vi "LEDColorControlRob.vi"(8 "error in":errorcluster) -> ()   [LabVIEW 2014]
uses:
  <vilib>/Rock Robotics/WPI/DriverStation/WPI_DriverStationRobotMode2.ctl
  <vilib>/Rock Robotics/WPI/Joystick/WPI_JoystickGetSetRefNum.vi
  Gantry/GantryGlobals.vi
  Robot Global Data.vi
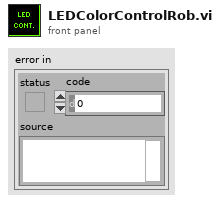
[diagram p1: front panel]
types:
  T1 = typedef "WPI_DriverStationRobotMode2.ctl" = enum16{"Autonomous Disabled", "Autonomous Enabled", "Teleop Disabled", "Teleop Enabled", "Disconnected", "Finish", "Test Disabled", "Test Enabled", "Emergency Stopped"}
  T2 = typedef "WPI_SPIDevRef.ctl" = cluster{"DevStatus":errorcluster, "Handle":i32, "Controller":T3, "SPI Bus":T4}
  T3 = typedef "FPGA_TypedefDigitalModule.ctl" = enum16{"Controller 1"}
  T4 = typedef "spi_bus.ctl" = enum16{"SPI On-Board, CS0", "SPI On-Board, CS1", "SPI On-Board, CS2", "SPI On-Board, CS3", "SPI MXP", "Invalid"}
  T5 = typedef "WPI_MotorControlDeviceRef.ctl" = cluster{"DeviceStatus":errorcluster, "Type":T6, "PWM":cluster{"Controller":T3, "PWM Channel":T7, "DeadBand":T8}, "CAN":cluster{"Device Number":u8, "Control Mode":T9, "Semaphore":T10, "Max Vout":dbl, "TalonSRX Control Mode":T11}, "Invert":bool, "TransformRef":T12, "InvTransformRef":T12}
  T6 = typedef "WPI_MotorControlType.ctl" = enum16{"PWM", "CAN", "CANTalonSRX"}
  T7 = typedef "FPGA_DIOPWMChannel.ctl" = enum8{"PWM 0", "PWM 1", "PWM 2", "PWM 3", "PWM 4", "PWM 5", "PWM 6", "PWM 7", "PWM 8", "PWM 9", "PWM MXP 0", "PWM MXP 1", "PWM MXP 2", "PWM MXP 3", "PWM MXP 4", "PWM MXP 5", "PWM MXP 6", "PWM MXP 7", "PWM MXP 8", "PWM MXP 9", "Invalid"}
  T8 = typedef "WPI_PWMDeadband.ctl" = cluster{"Name":string, "maxPositivePwm":i32, "minPositivePwm":i32, "centerPwm":i32, "maxNegativePwm":i32, "minNegativePwm":i32, "angularRange":u16}
  T9 = typedef "WPI_CANJaguar_ControlMode.ctl" = enum8{"Percent VBus", "Current", "Speed", "Position", "Voltage"}
  T10 = typedef "Semaphore RefNum" = refnum<k1>
  T11 = typedef "WPI_CANTalonSRX_APIControlMode.ctl" = enum8{"Percent VBus", "Speed", "Position", "Slave", "Unchanged / Invalid"}
  T12 = typedef "WPI_PWMTransform_ConPane.ctl" = refnum<vi>
  T13 = typedef "WPI_CANTalonSRX_GlobalStatus.ctl" = cluster{"Applied Throttle":dbl, "Module Enabled":bool, "CAN Error":errorcluster, "Closed Loop Error":dbl, "Forward Limit Switch Closed":bool, "Reverse Limit Switch Closed":bool, "Sensor Position":dbl, "Sensor Velocity":dbl, "Current":dbl, "Sticky Fault - Over Temp":bool, "Sticky Fault - Under Voltage":bool, "Sticky Fault - Forward Limit":bool, "Sticky Fault - Reverse Limit":bool, "Sticky Fault - Forward Soft Limit":bool, "Sticky Fault - Reverse Soft Limit":bool, "Brake is Enabled":bool, "Encoder Position":dbl, "Encoder Velocity":dbl, "Encoder Index Count":dbl, "Encoder A Pin State":bool, "Encoder B Pin State":bool, "Encoder Index Pin State":bool, "Analog In":dbl, "Analog In Velocity":dbl, "Temperature (C)":dbl, "Battery Voltage":dbl}
  T14 = typedef "WPI_JoystickDevRef.ctl" = cluster{"Device":T15}
  T15 = typedef "WPI_JoystickDeviceEnum.ctl" = enum16{"USB 0", "USB 1", "USB 2", "USB 3", "USB 4", "USB 5"}
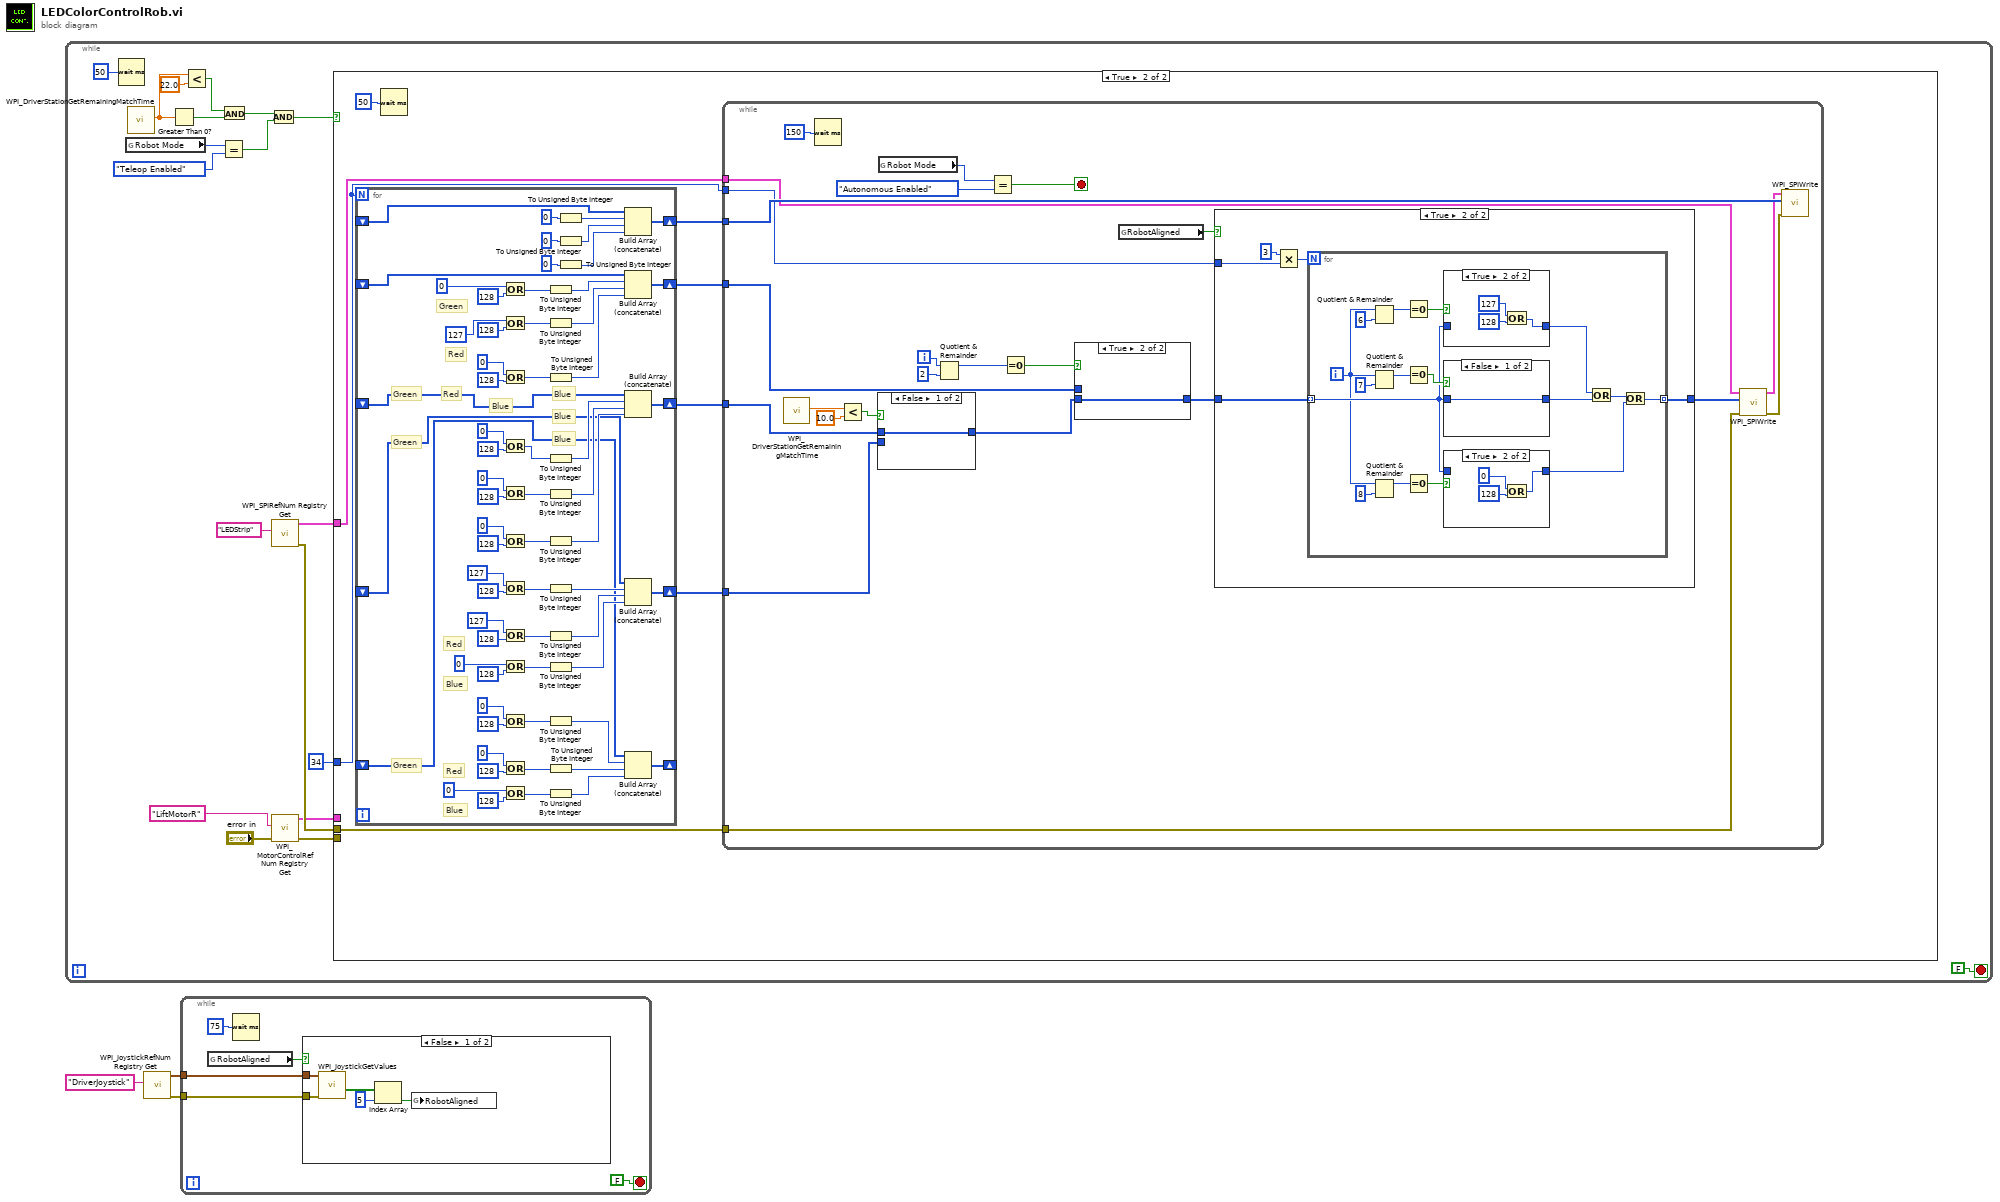
[diagram p0: block diagram]
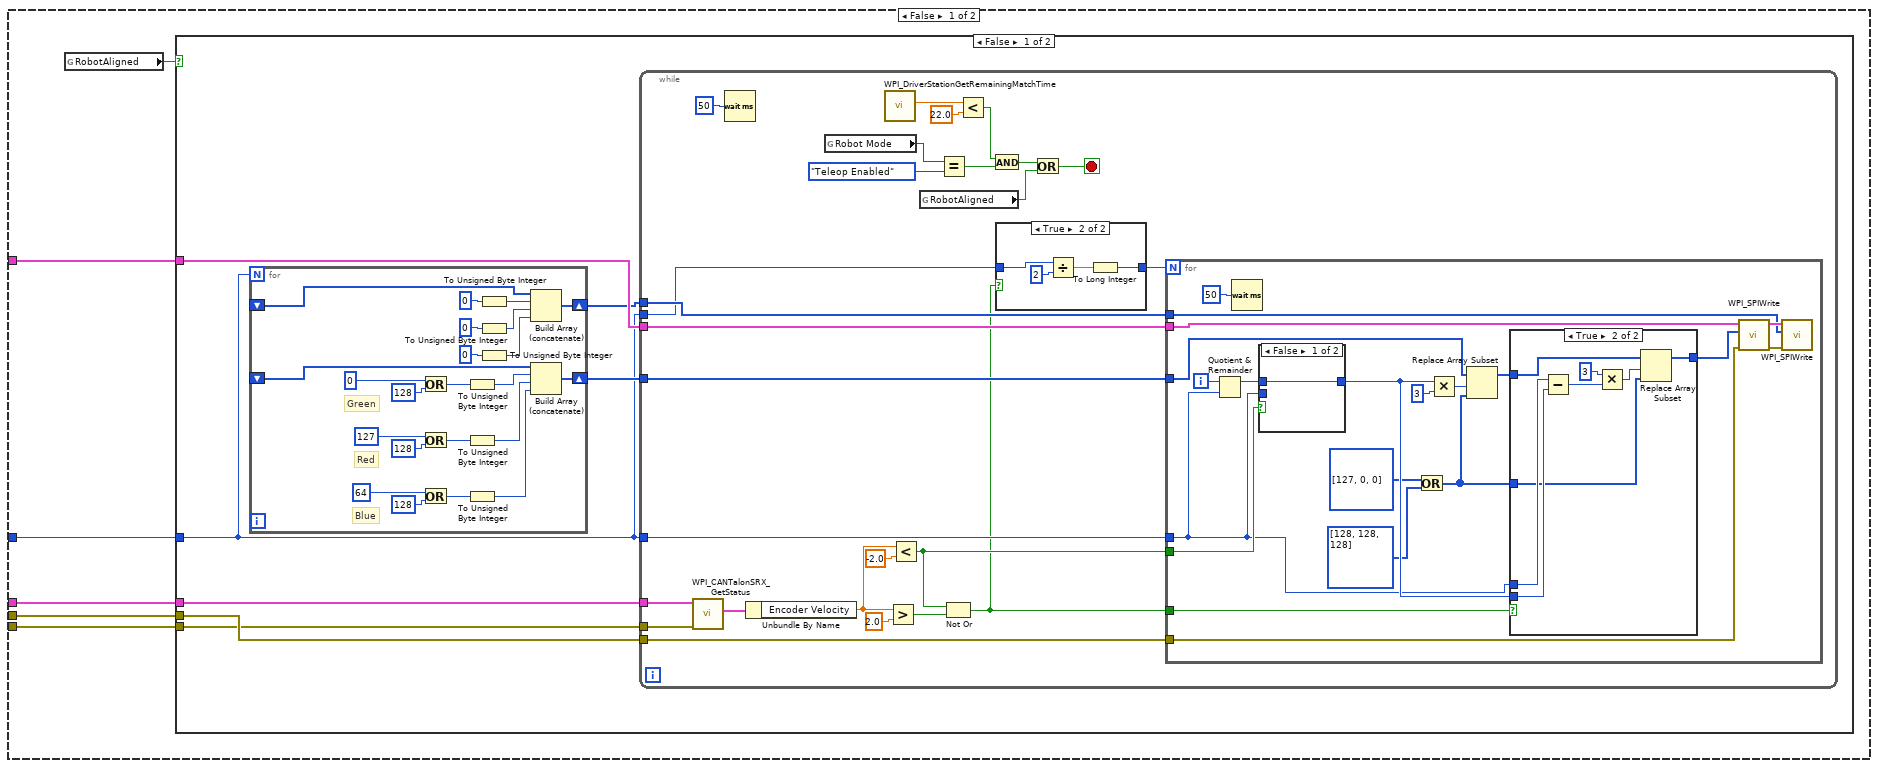
[diagram p2: hidden frame]
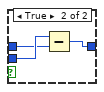
[diagram p5: hidden frame]
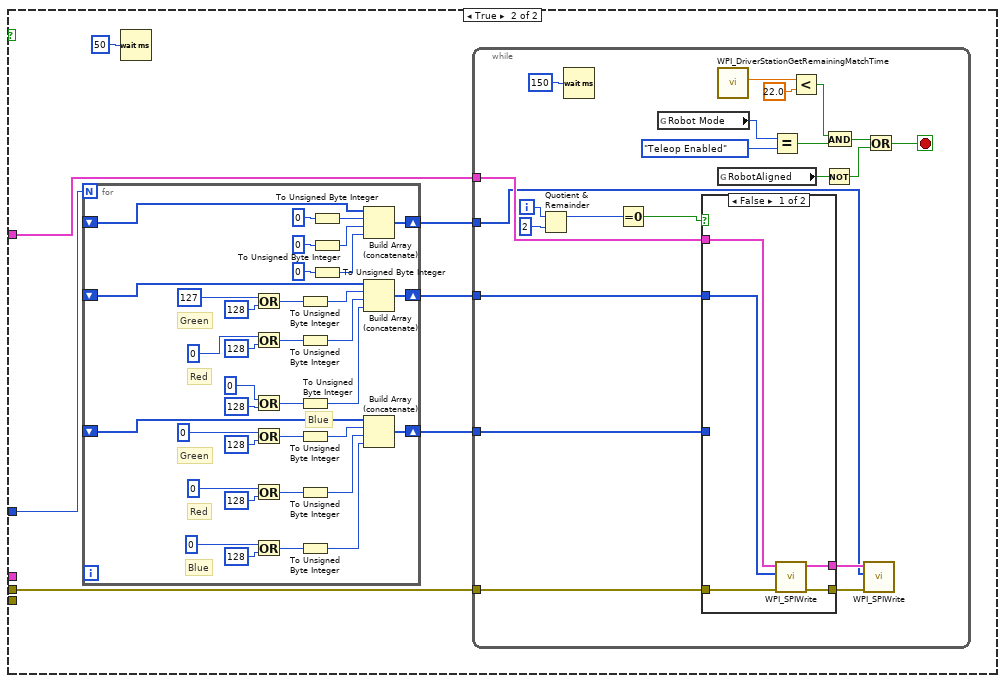
[diagram p6: hidden frame]
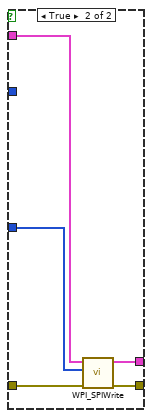
[diagram p7: hidden frame]
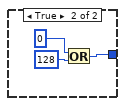
[diagram p10: hidden frame]
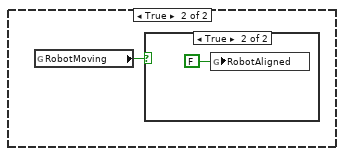
[diagram p14: hidden frame]
diagram:
  n1 = while {
    stop <- FALSE stop-if-true
    n2 = Wait (ms)(milliseconds to wait=u32 50) -> ()  [unwired: 1 out]
    n3 = global read "Robot Global Data.vi" "Robot Mode"() -> (w11:T1)
    n4 = call <vilib>:"WPI_DriverStationGetRemainingMatchTime.vi"() -> ("Match Time(s)"=w4:sgl)  [unwired: 10 in, 1 out]
    n5 = Greater Than 0?(x=w4) -> (x > 0?=w5:bool)
    n6 = Less?(x=w4, y=sgl 22.0) -> (x < y?=w8:bool)
    n7 = Equal?(x=w11, y=WPI_DriverStationRobotMode2."Teleop Enabled") -> (x = y?=w9:bool)
    n8 = And(x=w8, y=w5) -> (x .and. y?=w6:bool)
    n9 = And(x=w6, y=w9) -> (x .and. y?=w7:bool)
    n10 = call <vilib>:"WPI_SPIRefNum Registry Get.vi"("refnum name"="LEDStrip") -> ("error out"=w20:errorcluster, "SPIDevRef"=w21:T2)  [unwired: 9 in]
    n11 = call <vilib>:"WPI_MotorControlRefNum Registry Get.vi"("error in (no error)"="error in", "refnum name"="LiftMotorR") -> ("error out"=w15:errorcluster, "MotorControlDevRef"=w16:T5)  [unwired: 8 in]
    n12 = case shown="True" w7 {
      tunnel: w21 -> [w28 w204]
      tunnel: w20 -> [w27 w203]
      tunnel: 34 -> [w26 w197]
      tunnel: w16 -> [w25 _]
      tunnel: w15 -> [w24 _]
      frame False {
        n13 = global read "GantryGlobals.vi" "RobotAligned"() -> (w23:bool)
        n14 = case shown="False" w23 {
          tunnel: w28 -> [w35 w127]
          tunnel: w27 -> [w34 w126]
          tunnel: w26 -> [w31 w128]
          tunnel: w25 -> [w30 _]
          tunnel: w24 -> [w29 _]
          frame False {
            n15 = for {
              N: w31 -> [_]
              shift-right: [w121] -> w33
              shift-left: _ -> [w120]
              shift-right: [w110] -> w32
              shift-left: _ -> [w109]
              # "Blue"
              # "Red"
              # "Green"
              n16 = Or(x=0 ("y"), y=128) -> (x .or. y?=w105:i32)
              n17 = Or(x=127 ("y"), y=128) -> (x .or. y?=w106:i32)
              n18 = Or(x=64 ("y"), y=128) -> (x .or. y?=w107:i32)
              n19 = To Unsigned Byte Integer(number=w105) -> (unsigned 8bit integer=w119:u8)
              n20 = To Unsigned Byte Integer(number=w106) -> (unsigned 8bit integer=w118:u8)
              n21 = To Unsigned Byte Integer(number=w107) -> (unsigned 8bit integer=w117:u8)
              n22 = To Unsigned Byte Integer(number=0) -> (unsigned 8bit integer=w115:u8)
              n23 = To Unsigned Byte Integer(number=0) -> (unsigned 8bit integer=w114:u8)
              n24 = To Unsigned Byte Integer(number=0) -> (unsigned 8bit integer=w113:u8)
              n25 = Build Array (concatenate)(w109, w115, w114, w113) -> (w110:u8[])
              n26 = Build Array (concatenate)(w120, w119, w118, w117) -> (w121:u8[])
            }
            n27 = while {
              tunnel: w35 -> [w61]
              tunnel: w34 -> [w60]
              tunnel: w32 -> [w59]
              tunnel: w31 -> [w58]
              tunnel: w31 -> [w46]
              tunnel: w33 -> [w56]
              tunnel: w30 -> [w55]
              tunnel: w29 -> [w54]
              stop <- w41 stop-if-true
              n28 = call <vilib>:"WPI_CANTalonSRX_GetStatus.vi"("error in (no error)"=w54, "CAN Talon SRX Ref"=w55) -> ("Talon SRX Status"=w53:T13)  [unwired: 7 in, 2 out]
              n29 = Wait (ms)(milliseconds to wait=u32 50) -> ()  [unwired: 1 out]
              n30 = Unbundle By Name(w53) -> ("Encoder Velocity"=w51:dbl)
              n31 = global read "Robot Global Data.vi" "Robot Mode"() -> (w40:T1)
              n32 = call <vilib>:"WPI_DriverStationGetRemainingMatchTime.vi"() -> ("Match Time(s)"=w44:sgl)  [unwired: 10 in, 1 out]
              n33 = Greater?(x=w51, y=2.0) -> (0:w49:bool)
              n34 = Less?(x=w51, y=-2.0) -> (x < y?=w48:bool)
              n35 = global read "GantryGlobals.vi" "RobotAligned"() -> (w42:bool)
              n36 = Equal?(x=w40, y=WPI_DriverStationRobotMode2."Teleop Enabled") -> (x = y?=w38:bool)
              n37 = Not Or(1:w49, 2:w48) -> (0:w47:bool)
              n38 = Less?(x=w44, y=sgl 22.0) -> (x < y?=w37:bool)
              n39 = And(x=w37, y=w38) -> (x .and. y?=w36:bool)
              n40 = case shown="True" w47 {
                tunnel: w46 -> [w62 w66]
                tunnel: [w62 w63] -> w45
                frame False {
                }
                frame True {
                  n41 = Divide(x=w66, y=2) -> (x/y=w64:dbl)
                  n42 = To Long Integer(number=w64) -> (32bit integer=w63:i32)
                }
              }
              n43 = Or(x=w36, y=w42) -> (x .or. y?=w41:bool)
              n44 = for {
                N: w45 -> [_]
                tunnel: w61 -> [w84]
                tunnel: w60 -> [w83]
                tunnel: w59 -> [w81]
                tunnel: w58 -> [w70]
                tunnel: w56 -> [w79]
                tunnel: w48 -> [w75]
                tunnel: w47 -> [w72]
                i -> [w80]
                n45 = Quotient & Remainder(x=w80, y=w70) -> (x-y*floor(x/y)=w76:i32)  [unwired: 1 out]
                n46 = Wait (ms)(milliseconds to wait=u32 50) -> ()  [unwired: 1 out]
                n47 = case shown="False" w75 {
                  tunnel: w76 -> [w96 w98]
                  tunnel: [w96 w97] -> w71
                  tunnel: w70 -> [_ w99]
                  frame False {
                  }
                  frame True {
                    n48 = Subtract(x=w99, y=w98) -> (x-y=w97:i32)
                  }
                }
                n49 = Or(x=u8[] [127, 0, 0], y=u8[] [128, 128, 128]) -> (x .or. y?=w67:u8[])
                n50 = Multiply(x=w71, y=3) -> (x*y=w77:i32)
                n51 = Replace Array Subset(array=w79, new element=w67, index=w77) -> (w74:u8[])
                n52 = case shown="True" w72 {
                  tunnel: w74 -> [w87 w95]
                  tunnel: [w87 w94] -> w73
                  tunnel: w71 -> [_ w93]
                  tunnel: w70 -> [_ w92]
                  tunnel: w67 -> [_ w90]
                  frame False {
                  }
                  frame True {
                    n53 = Subtract(x=w92, y=w93) -> (x-y=w91:i32)
                    n54 = Multiply(x=3, y=w91) -> (x*y=w89:i32)
                    n55 = Replace Array Subset(array=w95, new element=w90, index=w89) -> (w94:u8[])
                  }
                }
                n56 = call <vilib>:"WPI_SPIWrite.vi"("error in (no error)"=w83, "Data To Send"=w73, "SPIDevRef"=w84) -> ("error out"=w82:errorcluster, "SPIDevRef"=w85:T2)  [unwired: 6 in, 1 out]
                n57 = call <vilib>:"WPI_SPIWrite.vi"("error in (no error)"=w82, "Data To Send"=w81, "SPIDevRef"=w85) -> ()  [unwired: 6 in, 3 out]
              }
            }
          }
          frame True {
            n58 = for {
              N: w128 -> [_]
              shift-right: [w196] -> w124
              shift-left: _ -> [w195]
              shift-right: [w185] -> w123
              shift-left: _ -> [w184]
              shift-right: [w162] -> w125
              shift-left: _ -> [w161]
              # "Blue"
              # "Red"
              # "Green"
              # "Blue"
              # "Red"
              # "Green"
              n59 = Or(x=127 ("y"), y=128) -> (x .or. y?=w180:i32)
              n60 = Or(x=0 ("y"), y=128) -> (x .or. y?=w181:i32)
              n61 = Or(x=0 ("y"), y=128) -> (x .or. y?=w182:i32)
              n62 = Or(x=0 ("y"), y=128) -> (x .or. y?=w168:i32)
              n63 = Or(x=0 ("y"), y=128) -> (x .or. y?=w169:i32)
              n64 = Or(x=0 ("y"), y=128) -> (x .or. y?=w170:i32)
              n65 = To Unsigned Byte Integer(number=w180) -> (unsigned 8bit integer=w194:u8)
              n66 = To Unsigned Byte Integer(number=w181) -> (unsigned 8bit integer=w193:u8)
              n67 = To Unsigned Byte Integer(number=w182) -> (unsigned 8bit integer=w192:u8)
              n68 = To Unsigned Byte Integer(number=w168) -> (unsigned 8bit integer=w174:u8)
              n69 = To Unsigned Byte Integer(number=w169) -> (unsigned 8bit integer=w173:u8)
              n70 = To Unsigned Byte Integer(number=w170) -> (unsigned 8bit integer=w172:u8)
              n71 = To Unsigned Byte Integer(number=0) -> (unsigned 8bit integer=w190:u8)
              n72 = To Unsigned Byte Integer(number=0) -> (unsigned 8bit integer=w189:u8)
              n73 = To Unsigned Byte Integer(number=0) -> (unsigned 8bit integer=w188:u8)
              n74 = Build Array (concatenate)(w184, w190, w189, w188) -> (w185:u8[])
              n75 = Build Array (concatenate)(w195, w194, w193, w192) -> (w196:u8[])
              n76 = Build Array (concatenate)(w161, w174, w173, w172) -> (w162:u8[])
            }
            n77 = Wait (ms)(milliseconds to wait=u32 50) -> ()  [unwired: 1 out]
            n78 = while {
              tunnel: w127 -> [w150]
              tunnel: w126 -> [w149]
              tunnel: w125 -> [w144]
              tunnel: w124 -> [w143]
              tunnel: w123 -> [w140]
              i -> [w148]
              stop <- w134 stop-if-true
              n79 = Quotient & Remainder(x=w148, y=2) -> (x-y*floor(x/y)=w146:i32)  [unwired: 1 out]
              n80 = Wait (ms)(milliseconds to wait=u32 150) -> ()  [unwired: 1 out]
              n81 = Equal To 0?(x=w146) -> (x = 0?=w145:bool)
              n82 = global read "Robot Global Data.vi" "Robot Mode"() -> (w133:T1)
              n83 = case shown="False" w145 {
                tunnel: w150 -> [w155 w160]
                tunnel: w149 -> [w154 w159]
                tunnel: w144 -> [_ w158]
                tunnel: w143 -> [w153 _]
                tunnel: [w152 w157] -> w142
                tunnel: [w151 w156] -> w141
                frame False {
                  n84 = call <vilib>:"WPI_SPIWrite.vi"("error in (no error)"=w154, "Data To Send"=w153, "SPIDevRef"=w155) -> ("error out"=w151:errorcluster, "SPIDevRef"=w152:T2)  [unwired: 6 in, 1 out]
                }
                frame True {
                  n85 = call <vilib>:"WPI_SPIWrite.vi"("error in (no error)"=w159, "Data To Send"=w158, "SPIDevRef"=w160) -> ("error out"=w156:errorcluster, "SPIDevRef"=w157:T2)  [unwired: 6 in, 1 out]
                }
              }
              n86 = call <vilib>:"WPI_DriverStationGetRemainingMatchTime.vi"() -> ("Match Time(s)"=w137:sgl)  [unwired: 10 in, 1 out]
              n87 = global read "GantryGlobals.vi" "RobotAligned"() -> (w139:bool)
              n88 = Equal?(x=w133, y=WPI_DriverStationRobotMode2."Teleop Enabled") -> (x = y?=w131:bool)
              n89 = Less?(x=w137, y=sgl 22.0) -> (x < y?=w130:bool)
              n90 = Not(x=w139) -> (.not. x?=w135:bool)
              n91 = And(x=w130, y=w131) -> (x .and. y?=w129:bool)
              n92 = call <vilib>:"WPI_SPIWrite.vi"("error in (no error)"=w141, "Data To Send"=w140, "SPIDevRef"=w142) -> ()  [unwired: 6 in, 3 out]
              n93 = Or(x=w129, y=w135) -> (x .or. y?=w134:bool)
            }
          }
        }
      }
      frame True {
        n94 = for {
          N: w197 -> [_]
          shift-right: [w330] -> w201
          shift-left: _ -> [w329]
          shift-right: [w319] -> w200
          shift-left: _ -> [w318]
          shift-right: [w296] -> w202
          shift-left: _ -> [w295]
          shift-right: [w282] -> w198
          shift-left: _ -> [w281]
          shift-right: [w268] -> _
          shift-left: _ -> [w267]
          # "Blue"
          # "Red"
          # "Green"
          # "Blue"
          # "Blue"
          # "Red"
          # "Green"
          # "Blue"
          # "Blue"
          # "Red"
          # "Green"
          # "Blue"
          # "Red"
          # "Green"
          n95 = Or(x=0 ("y"), y=128) -> (x .or. y?=w314:i32)
          n96 = Or(x=127 ("y"), y=128) -> (x .or. y?=w315:i32)
          n97 = Or(x=0 ("y"), y=128) -> (x .or. y?=w316:i32)
          n98 = Or(x=0 ("y"), y=128) -> (x .or. y?=w302:i32)
          n99 = Or(x=0 ("y"), y=128) -> (x .or. y?=w303:i32)
          n100 = Or(x=0 ("y"), y=128) -> (x .or. y?=w304:i32)
          n101 = Or(x=127 ("y"), y=128) -> (x .or. y?=w288:i32)
          n102 = Or(x=127 ("y"), y=128) -> (x .or. y?=w289:i32)
          n103 = Or(x=0 ("y"), y=128) -> (x .or. y?=w290:i32)
          n104 = Or(x=0 ("y"), y=128) -> (x .or. y?=w274:i32)
          n105 = Or(x=0 ("y"), y=128) -> (x .or. y?=w275:i32)
          n106 = Or(x=0 ("y"), y=128) -> (x .or. y?=w276:i32)
          n107 = To Unsigned Byte Integer(number=w314) -> (unsigned 8bit integer=w328:u8)
          n108 = To Unsigned Byte Integer(number=w315) -> (unsigned 8bit integer=w327:u8)
          n109 = To Unsigned Byte Integer(number=w316) -> (unsigned 8bit integer=w326:u8)
          n110 = To Unsigned Byte Integer(number=w302) -> (unsigned 8bit integer=w308:u8)
          n111 = To Unsigned Byte Integer(number=w303) -> (unsigned 8bit integer=w307:u8)
          n112 = To Unsigned Byte Integer(number=w304) -> (unsigned 8bit integer=w306:u8)
          n113 = To Unsigned Byte Integer(number=w288) -> (unsigned 8bit integer=w294:u8)
          n114 = To Unsigned Byte Integer(number=w289) -> (unsigned 8bit integer=w293:u8)
          n115 = To Unsigned Byte Integer(number=w290) -> (unsigned 8bit integer=w292:u8)
          n116 = To Unsigned Byte Integer(number=w274) -> (unsigned 8bit integer=w280:u8)
          n117 = To Unsigned Byte Integer(number=w275) -> (unsigned 8bit integer=w279:u8)
          n118 = To Unsigned Byte Integer(number=w276) -> (unsigned 8bit integer=w278:u8)
          n119 = To Unsigned Byte Integer(number=0) -> (unsigned 8bit integer=w324:u8)
          n120 = To Unsigned Byte Integer(number=0) -> (unsigned 8bit integer=w323:u8)
          n121 = To Unsigned Byte Integer(number=0) -> (unsigned 8bit integer=w322:u8)
          n122 = Build Array (concatenate)(w318, w324, w323, w322) -> (w319:u8[])
          n123 = Build Array (concatenate)(w329, w328, w327, w326) -> (w330:u8[])
          n124 = Build Array (concatenate)(w295, w308, w307, w306) -> (w296:u8[])
          n125 = Build Array (concatenate)(w281, w294, w293, w292) -> (w282:u8[])
          n126 = Build Array (concatenate)(w267, w280, w279, w278) -> (w268:u8[])
        }
        n127 = Wait (ms)(milliseconds to wait=u32 50) -> ()  [unwired: 1 out]
        n128 = while {
          tunnel: w204 -> [w211]
          tunnel: w203 -> [w210]
          tunnel: w202 -> [w218]
          tunnel: w201 -> [w224]
          tunnel: w200 -> [w223]
          tunnel: w198 -> [w217]
          tunnel: w197 -> [w213]
          i -> [w228]
          stop <- w214 stop-if-true
          n129 = call <vilib>:"WPI_DriverStationGetRemainingMatchTime.vi"() -> ("Match Time(s)"=w221:sgl)  [unwired: 10 in, 1 out]
          n130 = Wait (ms)(milliseconds to wait=u32 150) -> ()  [unwired: 1 out]
          n131 = Less?(x=w221, y=sgl 10.0) -> (x < y?=w219:bool)
          n132 = case shown="False" w219 {
            tunnel: w218 -> [w263 _]
            tunnel: w217 -> [_ w264]
            tunnel: [w263 w264] -> w209
            frame False {
            }
            frame True {
            }
          }
          n133 = global read "Robot Global Data.vi" "Robot Mode"() -> (w216:T1)
          n134 = Quotient & Remainder(x=w228, y=2) -> (x-y*floor(x/y)=w226:i32)  [unwired: 1 out]
          n135 = Equal?(x=w216, y=WPI_DriverStationRobotMode2."Autonomous Enabled") -> (x = y?=w214:bool)
          n136 = Equal To 0?(x=w226) -> (x = 0?=w225:bool)
          n137 = case shown="True" w225 {
            tunnel: w224 -> [w265 _]
            tunnel: w209 -> [_ w266]
            tunnel: [w265 w266] -> w205
            frame False {
            }
            frame True {
            }
          }
          n138 = global read "GantryGlobals.vi" "RobotAligned"() -> (w212:bool)
          n139 = case shown="True" w212 {
            tunnel: w213 -> [_ w234]
            tunnel: [w229 w231] -> w206
            tunnel: w205 -> [w229 w230]
            frame False {
            }
            frame True {
              n140 = Multiply(x=3, y=w234) -> (x*y=w233:i32)
              n141 = for {
                N: w233 -> [_]
                tunnel: [w236] -> w231 mode=indexing
                tunnel: w230 -> [w241] mode=indexing
                i -> [w235]
                n142 = Quotient & Remainder(x=w235, y=6) -> (x-y*floor(x/y)=w249:i32)  [unwired: 1 out]
                n143 = Quotient & Remainder(x=w235, y=7) -> (x-y*floor(x/y)=w246:i32)  [unwired: 1 out]
                n144 = Quotient & Remainder(x=w235, y=8) -> (x-y*floor(x/y)=w243:i32)  [unwired: 1 out]
                n145 = Equal To 0?(x=w249) -> (x = 0?=w248:bool)
                n146 = Equal To 0?(x=w246) -> (x = 0?=w245:bool)
                n147 = Equal To 0?(x=w243) -> (x = 0?=w242:bool)
                n148 = case shown="True" w248 {
                  tunnel: [w259 w262] -> w240
                  tunnel: w241 -> [w259 _]
                  frame False {
                  }
                  frame True {
                    n149 = Or(x=u8 127, y=u8 128) -> (x .or. y?=w262:u8)
                  }
                }
                n150 = case shown="False" w245 {
                  tunnel: [w255 w258] -> w239
                  tunnel: w241 -> [w255 _]
                  frame False {
                  }
                  frame True {
                    n151 = Or(x=u8 0, y=u8 128) -> (x .or. y?=w258:u8)
                  }
                }
                n152 = case shown="True" w242 {
                  tunnel: [w251 w254] -> w237
                  tunnel: w241 -> [w251 _]
                  frame False {
                  }
                  frame True {
                    n153 = Or(x=u8 0, y=u8 128) -> (x .or. y?=w254:u8)
                  }
                }
                n154 = Or(x=w240, y=w239) -> (x .or. y?=w238:u8)
                n155 = Or(x=w238, y=w237) -> (x .or. y?=w236:u8)
              }
            }
          }
          n156 = call <vilib>:"WPI_SPIWrite.vi"("error in (no error)"=w210, "Data To Send"=w206, "SPIDevRef"=w211) -> ("error out"=w207:errorcluster, "SPIDevRef"=w208:T2)  [unwired: 6 in, 1 out]
          n157 = call <vilib>:"WPI_SPIWrite.vi"("error in (no error)"=w207, "Data To Send"=w223, "SPIDevRef"=w208) -> ()  [unwired: 6 in, 3 out]
        }
      }
    }
  }
  n158 = call <vilib>:"WPI_JoystickRefNum Registry Get.vi"("refnum name"="DriverJoystick") -> ("error out"=w1:errorcluster, "JoystickDevRef"=w2:T14)  [unwired: 9 in]
  n159 = while {
    tunnel: w2 -> [w332]
    tunnel: w1 -> [w331]
    stop <- FALSE stop-if-true
    n160 = global read "GantryGlobals.vi" "RobotAligned"() -> (w334:bool)
    n161 = Wait (ms)(milliseconds to wait=u32 75) -> ()  [unwired: 1 out]
    n162 = case shown="False" w334 {
      tunnel: w332 -> [w339 _]
      tunnel: w331 -> [w338 _]
      frame False {
        n163 = call <vilib>:"WPI_JoystickGetValues.vi"("error in (no error)"=w338, "JoystickDevRef"=w339) -> ("Buttons"=w337:bool[])  [unwired: 5 in, 4 out]
        n164 = Index Array(array=w337, index=5) -> (element=w336:bool)
        n165 = global write "GantryGlobals.vi" "RobotAligned"(w336) -> ()
      }
      frame True {
        n166 = global read "GantryGlobals.vi" "RobotMoving"() -> (w341:bool)
        n167 = case shown="True" w341 {
          frame False {
          }
          frame True {
            n168 = global write "GantryGlobals.vi" "RobotAligned"(FALSE ("RobotAligned")) -> ()
          }
        }
      }
    }
  }
